vi "Time Step.vi"(11 "Snake in":refnum<class "Snake.lvclass">) -> (3 "Snake out":refnum<class "Snake.lvclass">)   [LabVIEW 2020, in "Snake.lvclass"]
uses:
  Snake.lvclass
  Snake.lvclass/Snake.ctl
  Particle.lvclass/Particle.ctl
  Particle.lvclass
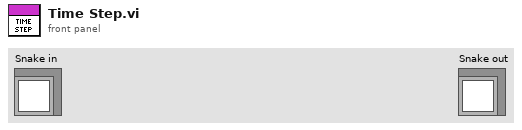
[diagram p1: front panel]
types:
  T1 = typedef "Direction.ctl" = enum16{"X", "-X", "Y", "-Y"}
  T2 = typedef "Particle.lvclass/Position.ctl" = cluster{"X":i32, "Y":i32}
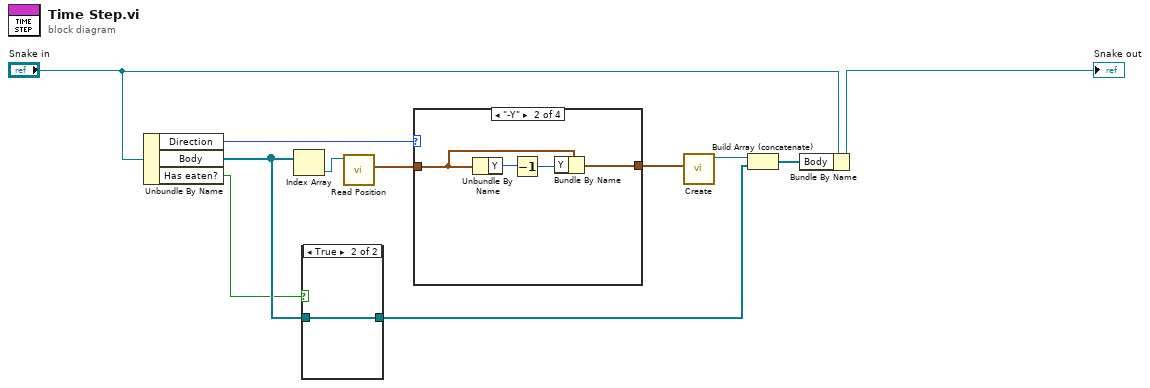
[diagram p0: block diagram]
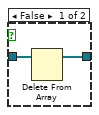
[diagram p2: hidden frame]
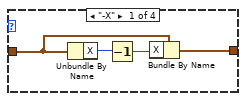
[diagram p3: hidden frame]
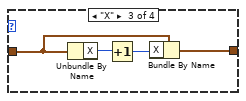
[diagram p4: hidden frame]
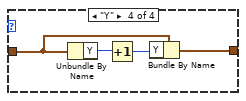
[diagram p5: hidden frame]
diagram:
  n1 = Unbundle By Name("Snake in") -> ("Direction"=w9:T1, "Body"=w5:refnum<class "Particle.lvclass">[], "Has eaten?"=w1:bool)
  n2 = Index Array(array=w5) -> (element=w4:refnum<class "Particle.lvclass">)  [unwired: 1 in]
  n3 = case shown="True" w1 {
    tunnel: w5 -> [w13 w14]
    tunnel: [w12 w14] -> w2
    frame False {
      n4 = Delete From Array(array=w13) -> (array with subset deleted=w12:refnum<class "Particle.lvclass">[])  [unwired: 2 in, 1 out]
    }
    frame True {
    }
  }
  n5 = call "Read Position.vi"("Particle in"=w4) -> ("Position"=w8:T2)  [unwired: 9 in, 1 out]
  n6 = case shown="\"-Y\"" w9 {
    tunnel: w8 -> [w17 w21 w25 w29]
    tunnel: [w15 w19 w23 w27] -> w7
    frame "-X" {
      n7 = Unbundle By Name(w17) -> ("X"=w18:i32)
      n8 = Decrement(x=w18) -> (x-1=w16:i32)
      n9 = Bundle By Name(cluster=w17, "X"=w16) -> (w15:T2)
    }
    frame "-Y" {
      n10 = Unbundle By Name(w21) -> ("Y"=w22:i32)
      n11 = Decrement(x=w22) -> (x-1=w20:i32)
      n12 = Bundle By Name(cluster=w21, "Y"=w20) -> (w19:T2)
    }
    frame "X" {
      n13 = Unbundle By Name(w25) -> ("X"=w26:i32)
      n14 = Increment(x=w26) -> (x+1=w24:i32)
      n15 = Bundle By Name(cluster=w25, "X"=w24) -> (w23:T2)
    }
    frame "Y" {
      n16 = Unbundle By Name(w29) -> ("Y"=w30:i32)
      n17 = Increment(x=w30) -> (x+1=w28:i32)
      n18 = Bundle By Name(cluster=w29, "Y"=w28) -> (w27:T2)
    }
  }
  n19 = call "Create.vi"("Position"=w7) -> ("Particle out"=w6:refnum<class "Particle.lvclass">)  [unwired: 10 in]
  n20 = Build Array (concatenate)(w6, w2) -> (w3:refnum<class "Particle.lvclass">[])
  n21 = Bundle By Name(cluster="Snake in", "Body"=w3) -> (→"Snake out":refnum<class "Snake.lvclass">)
